vi "Query Sequencer ARB File All Reliability Messages.vi"(8 "error in (no error)":errorcluster, 10 "Instance (1)":i32=1, 11 "VISA resource name":refnum<visa-resource-name>) -> (0 "error out":errorcluster, 2 "Reliability Messages":string, 3 "VISA resource name out":refnum<visa-resource-name>)   [LabVIEW 2015, in "Rohde&Schwarz CMXP GPRF.lvlib"]
doc: "Queries the reliability messages of all ARB files.\n\nAttribute:\nRSCMXPGPRF_ATTR_SEQUENCER_ARB_FILE_ALL_RELIABILITY_MESSAGES\n\nRemote-control command:\nSOURce:GPRF:GEN<i>:SEQuencer:APOol:RMESsage:ALL?"
uses:
  <instrlib>/Rohde&Schwarz CMXP GPRF/Rohde&Schwarz CMXP GPRF.lvlib
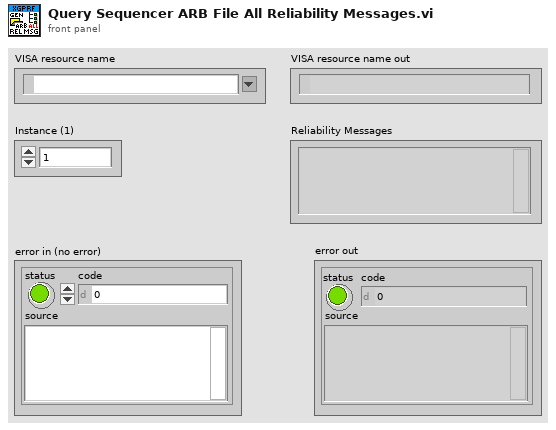
[diagram p1: front panel]
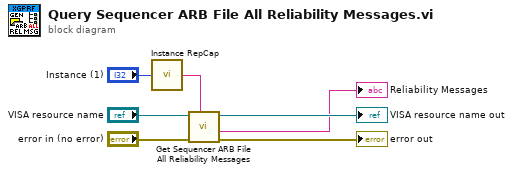
[diagram p0: block diagram]
diagram:
  n1 = call <instrlib>:"Instance RepCap.vi"("instance  in"="Instance (1)") -> ("instance out"=w2:string)
  n2 = call "Get Sequencer ARB File All Reliability Messages"("Repeated Capabilities"=w2, "error in (no error)"="error in (no error)", "instrument handle"="VISA resource name") -> ("error out"=→"error out":errorcluster, "Sequencer ARB File All Reliability Messages"=→"Reliability Messages":string, "instrument handle out"=→"VISA resource name out":refnum<visa-resource-name>)  [unwired: 6 in]
